vi "MIMICProtocol.vi"(4 "Input_Data":string[](array[string]), 5 "Error In":errorcluster, 6 "RSP_DelayTime":dbl caption="Delay Time (s)", 7 "ACK_DelayTime":dbl caption="Delay Time (s)", 8 "MIMIC_Command":string) -> (0 "Error Out":errorcluster, 1 "Status":bool, 2 "RESPONSE_Buffer":u8[](array[numeric]) format="%x", 3 "Generic_Mimic_Data 2":T1)   [LabVIEW 2014]
uses:
  Responses/MIMIC_ResponseCluster.ctl
panel:
  out "Validate \nCheckSum":bool
  out "ACK/NAK_Buffer":u8[](array[numeric])=[0, 0, 0, 0, 0, 0, 69, 83, 84, 32, 67, 79, 77, 80, 76, 69, 84, 69, 13, 10, 251, 226, 0, 0, 0, 0, 0, 0, 0, 0, 0, 0, 0, 0, 0, 0, 0, 0, 0, 0, 0, 0, 0, 0, 0, 0, 0, 0, 0, 0, 0, 0, 0, 0, 0, 0, 0, 0, 0, 0, 0, 0, 0, 0, 0, 0, 0, 0, 0, 0, 0, 0, 0, 0, 0, 0, 0, 0, 0, 0, 0, 0, 0, 0, 0, 0, 0, 0, 0, 0, 0, 0, 0, 0, 0, 0, 0, 0, 0, 0, 0, 0, 0, 0, 0, 0, 0, 0, 0, 0, 0, 0, 0, 0, 0, 0, 0, 0, 0, 0, 0, 0, 0, 0, 0, 0, 0, 0, 0, 0, 0, 0, 0, 0, 0, 0, 0, 0, 0, 0, 0, 0, 0, 0, 0, 0, 0, 0, 0, 0, 0, 0, 0, 0, 0, 0, 0, 0, 0, 0, 0, 0, 0, 0, 0, 0, 0, 0, 0, 0, 0, 0, 0, 0, 0, 0, 0, 0, 0, 0, 0, 0, 0, 0, 0, 0, 0, 0, 0, 0, 0, 0, 0, 0, 0, 0, 0, 0, 0, 0, 0, 0, 0, 0, 0, 0, 0, 0, 0, 0, 0, 0, 0, 0, 0, 0, 0, 0, 0, 0, 0, 0, 0, 0, 0, 0, 0, 0, 0, 0, 0, 0, 0, 0, 0, 0, 0, 0, 0, 0, 0, 0, 0, 0, 0, 0, 0, 0, 0, 0, 0, 0, 0, 0, 0, 0, 0, 0, 0, 0, 0, 0, 0, 0, 0, 0, 0, 0, 0, 0, 0, 0, 0, 0, 0, 0, 0] format="%x"
  in  "RSP_MimicProtocol VI Refnum":refnum<vi>
  out "Add \nChecksum":bool
  in  "CMD_MimicProtocol VI Refnum":refnum<vi>
  out "Send \nCommand":bool
  out "Command\n Sent":bool
  out "Response\n Received":bool
  out "ACK \nReceived":bool
  out "Check \nACK/NAK":bool
  out "Command":u8[](array[numeric]) format="%x"
  out "Obtain \nResponse":bool
  # "Outputs"
  # "Inputs"
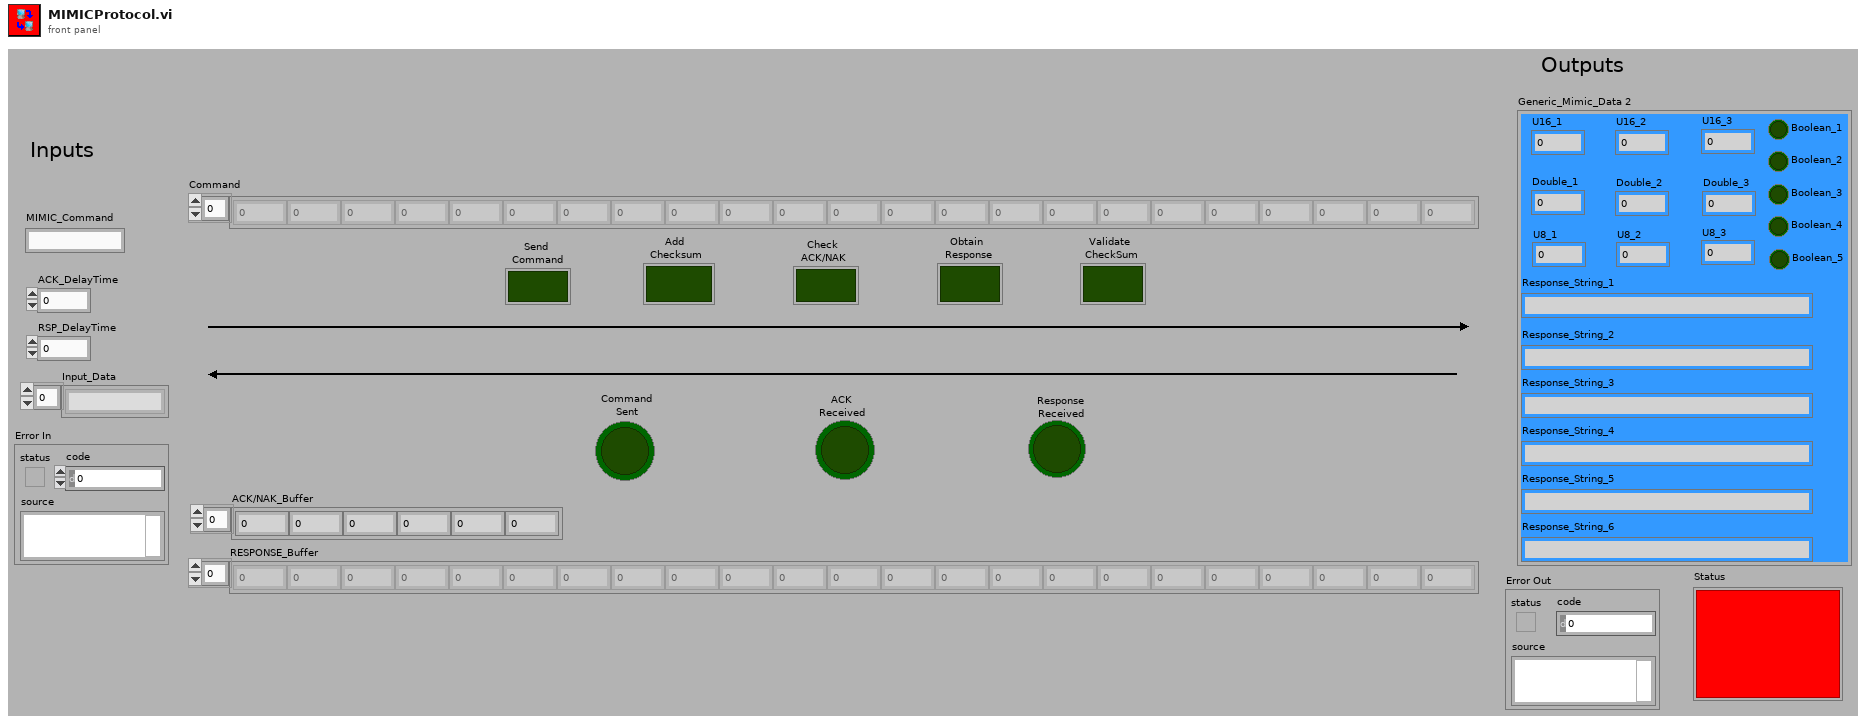
[diagram p1: front panel]
types:
  T1 = typedef "MIMIC_ResponseCluster.ctl" = cluster{"Response_String_1":string, "Response_String_2":string, "Response_String_3":string, "Response_String_4":string, "Response_String_5":string, "Response_String_6":string, "U16_1":u16, "Boolean_1":bool, "Boolean_2":bool, "Boolean_3":bool, "Boolean_4":bool, "Boolean_5":bool, "U16_2":u16, "U16_3":u16, "Double_1":dbl, "Double_2":dbl, "Double_3":dbl, "U8_1":dbl, "U8_2":dbl, "U8_3":dbl}
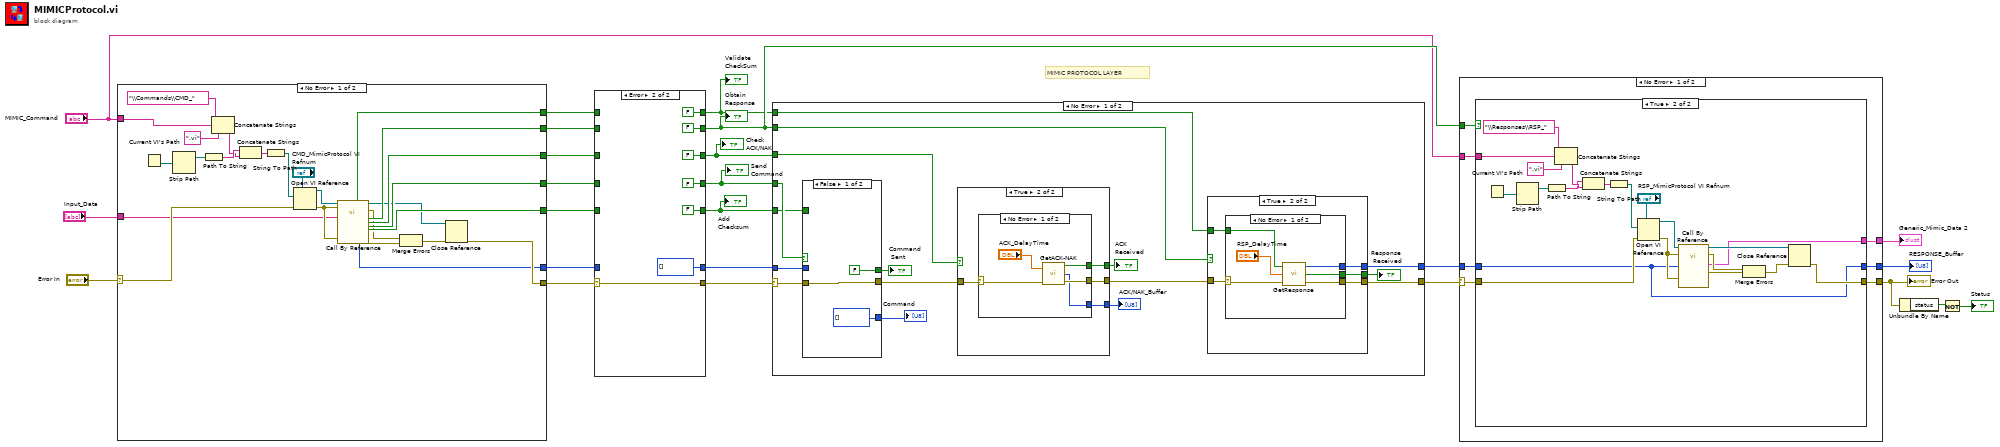
[diagram p0: block diagram]
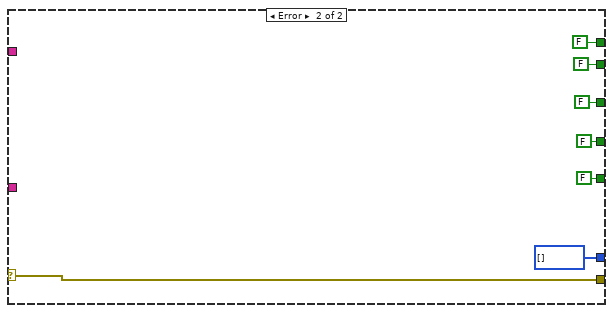
[diagram p3: hidden frame]
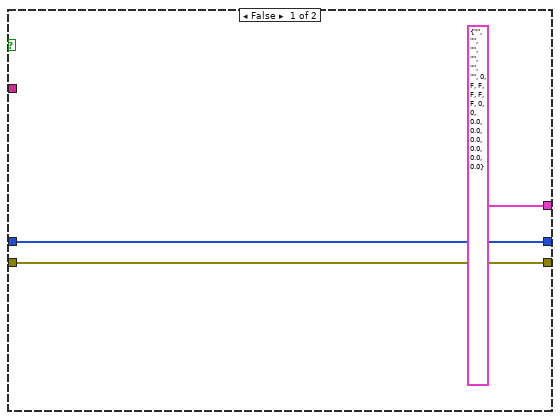
[diagram p4: hidden frame]
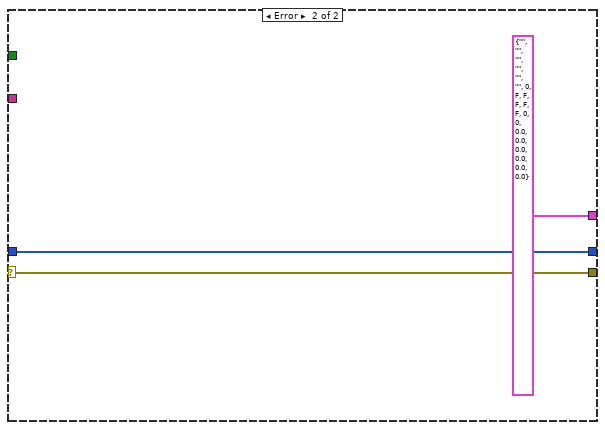
[diagram p5: hidden frame]
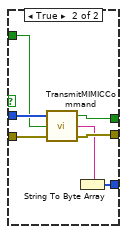
[diagram p6: hidden frame]
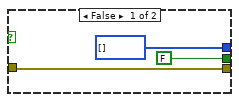
[diagram p7: hidden frame]
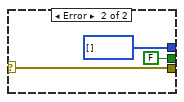
[diagram p8: hidden frame]
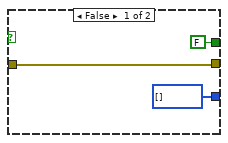
[diagram p9: hidden frame]
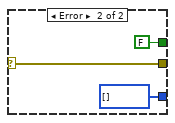
[diagram p10: hidden frame]
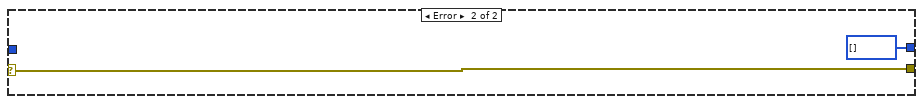
[diagram p11: hidden frame]
diagram:
  # "MIMIC PROTOCOL LAYER"
  n1 = case shown="No Error" "Error In" {
    selector: "Error In" -> [w48 w56]
    tunnel: [w43 w56] -> w12
    tunnel: "MIMIC_Command" -> [w46 _]
    tunnel: "Input_Data" -> [w34 _]
    tunnel: [w30 FALSE ("Command")] -> w16
    tunnel: [w31 FALSE ("Ack")] -> w18
    tunnel: [w32 FALSE ("Response")] -> w19
    tunnel: [w29 FALSE ("CheckSum")] -> w14
    tunnel: [w25 u8[] [] ("Command")] -> w10
    tunnel: [w28 FALSE ("Validate CheckSum")] -> w2
    frame No Error {
      n2 = Current VI's Path() -> (path=w49:path)
      n3 = Strip Path(path=w49) -> (stripped path=w42:path)  [unwired: 1 out]
      n4 = Path To String(path=w42) -> (string=w39:string)
      n5 = Concatenate Strings("\\Commands\\CMD_" ("string"), w46, ".vi" ("string")) -> (w38:string)
      n6 = Concatenate Strings(w39, w38) -> (w41:string)
      n7 = String To Path(string=w41) -> (path=w40:path)
      n8 = Open VI Reference(type specifier VI Refnum (for type only)="CMD_MimicProtocol VI Refnum", vi path=w40, error in (no error)=w48) -> (vi reference=w36:refnum<vi>, error out=w35:errorcluster)  [unwired: 3 in]
      n9 = call-by-ref "?"(reference=w36, error in=w35, "Input_Data"=w34, "Error In"=w35) -> (reference out=w26:refnum<vi>, error out=w27:errorcluster, "Validate CheckSum"=w28:bool, 13:"Command"=w25:u8[], "Response"=w32:bool, "Ack"=w31:bool, 16:"Command"=w30:bool, "Add CheckSum"=w29:bool, "Error Out"=w33:errorcluster)  [unwired: 10 in, 1 out]
      n10 = Merge Errors(w27, w33) -> (w44:errorcluster)
      n11 = Close Reference(reference=w26, error in (no error)=w44) -> (error out=w43:errorcluster)
    }
    frame Error {
    }
  }
  n12 = case shown="Error" w12 {
    selector: w12 -> [w59 w65]
    tunnel: [w63 FALSE ("Response")] -> w20
    tunnel: w19 -> [w63 _]
    tunnel: [w62 FALSE ("Ack")] -> w17
    tunnel: w18 -> [w62 _]
    tunnel: [w61 FALSE ("Command")] -> w15
    tunnel: w16 -> [w61 _]
    tunnel: [w60 FALSE ("CheckSum")] -> w13
    tunnel: w14 -> [w60 _]
    tunnel: [w59 w65] -> w11
    tunnel: [w58 u8[] [] ("Command")] -> w9
    tunnel: w10 -> [w58 _]
    tunnel: w2 -> [w57 _]
    tunnel: [w57 FALSE ("Validate CheckSum")] -> w1
    frame No Error {
    }
    frame Error {
    }
  }
  "Obtain \nResponse" <- w20
  "Check \nACK/NAK" <- w17
  "Send \nCommand" <- w15
  "Add \nChecksum" <- w13
  "Validate \nCheckSum" <- w1
  n13 = case shown="No Error" w11 {
    selector: w11 -> [w82 w130]
    tunnel: [w86 w130] -> w24
    tunnel: [w85 u8[] [] ("Receive_buffer out")] -> w23
    tunnel: w17 -> [w78 _]
    tunnel: w20 -> [w74 _]
    tunnel: w9 -> [w81 _]
    tunnel: w15 -> [w76 _]
    tunnel: w13 -> [w75 _]
    tunnel: w1 -> [w71 _]
    frame No Error {
      n14 = case shown="False" w76 {
        tunnel: [w89 w96] -> w84
        tunnel: w82 -> [w89 w95]
        tunnel: w81 -> [_ w94]
        tunnel: [FALSE ("Status") w93] -> w77
        tunnel: w75 -> [_ w92]
        tunnel: [u8[] [] ("unsigned byte array") w90] -> w72
        frame False {
        }
        frame True {
          n15 = call "TransmitMIMICCommand.vi"("Error In"=w95, "CheckSum?"=w92, "Command array"=w94) -> ("Error Out"=w96:errorcluster, "MIMIC_CMD"=w91:string, "Status"=w93:bool)
          n16 = String To Byte Array(string=w91) -> (unsigned byte array=w90:u8[])
        }
      }
      "Command\n Sent" <- w77
      "Command" <- w72
      n17 = case shown="True" w78 {
        tunnel: w84 -> [w116 w118]
        tunnel: [w116 w120] -> w83
        tunnel: [FALSE ("Status") w119] -> w80
        tunnel: [u8[] [] ("Receive_buffer") w117] -> w73
        frame False {
        }
        frame True {
          n18 = case shown="No Error" w118 {
            selector: w118 -> [w122 w128]
            tunnel: [w125 w128] -> w120
            tunnel: [w123 FALSE ("Status")] -> w119
            tunnel: [w121 u8[] [] ("Receive_buffer")] -> w117
            frame No Error {
              n19 = call "GetACK-NAK.vi"("error in"=w122, "Delay Time (s)"="ACK_DelayTime") -> ("error out"=w125:errorcluster, "Receive_buffer"=w121:u8[], "Status"=w123:bool)
            }
            frame Error {
            }
          }
        }
      }
      "ACK \nReceived" <- w80
      "ACK/NAK_Buffer" <- w73
      n20 = case shown="True" w74 {
        tunnel: [w99 w104] -> w86
        tunnel: [u8[] [] ("Receive_buffer out") w103] -> w85
        tunnel: w83 -> [w99 w101]
        tunnel: [FALSE ("Status") w102] -> w79
        tunnel: w71 -> [_ w100]
        frame False {
        }
        frame True {
          n21 = case shown="No Error" w101 {
            selector: w101 -> [w106 w113]
            tunnel: [w110 w113] -> w104
            tunnel: [w109 u8[] [] ("Receive_buffer out")] -> w103
            tunnel: [w107 FALSE ("Status")] -> w102
            tunnel: w100 -> [w105 _]
            frame No Error {
              n22 = call "GetResponse.vi"("error in"=w106, "Delay Time (s)"="RSP_DelayTime", "Validate Checksum"=w105) -> ("error out"=w110:errorcluster, "Status"=w107:bool, "Receive_buffer out"=w109:u8[])
            }
            frame Error {
            }
          }
        }
      }
      "Response\n Received" <- w79
    }
    frame Error {
    }
  }
  n23 = case shown="No Error" w24 {
    selector: w24 -> [w135 w162]
    tunnel: w23 -> [w136 w163]
    tunnel: w20 -> [w137 _]
    tunnel: [w134 w162] -> w7
    tunnel: [w133 w163] -> w8
    tunnel: "MIMIC_Command" -> [w132 _]
    tunnel: [w131 T1 {"Response_String_1"="", "Response_String_2"="", "Response_String_3"="", "Response_String_4"="", "Response_String_5"="", "Response_String_6"="", "U16_1"=0, "Boolean_1"=FALSE, "Boolean_2"=FALSE, "Boolean_3"=FALSE, "Boolean_4"=FALSE, "Boolean_5"=FALSE, "U16_2"=0, "U16_3"=0, "Double_1"=0.0, "Double_2"=0.0, "Double_3"=0.0, "U8_1"=0.0, "U8_2"=0.0, "U8_3"=0.0} ("Generic_Mimic_Data")] -> w3
    frame No Error {
      n24 = case shown="True" w137 {
        tunnel: w136 -> [w140 w142]
        tunnel: [w140 w142] -> w133
        tunnel: w135 -> [w139 w148]
        tunnel: [w139 w143] -> w134
        tunnel: w132 -> [_ w151]
        tunnel: [T1 {"Response_String_1"="", "Response_String_2"="", "Response_String_3"="", "Response_String_4"="", "Response_String_5"="", "Response_String_6"="", "U16_1"=0, "Boolean_1"=FALSE, "Boolean_2"=FALSE, "Boolean_3"=FALSE, "Boolean_4"=FALSE, "Boolean_5"=FALSE, "U16_2"=0, "U16_3"=0, "Double_1"=0.0, "Double_2"=0.0, "Double_3"=0.0, "U8_1"=0.0, "U8_2"=0.0, "U8_3"=0.0} ("Generic_Mimic_Data") w141] -> w131
        frame False {
        }
        frame True {
          n25 = Current VI's Path() -> (path=w152:path)
          n26 = Strip Path(path=w152) -> (stripped path=w156:path)  [unwired: 1 out]
          n27 = Path To String(path=w156) -> (string=w159:string)
          n28 = Concatenate Strings("\\Responses\\RSP_" ("string"), w151, ".vi" ("string")) -> (w160:string)
          n29 = Concatenate Strings(w159, w160) -> (w157:string)
          n30 = String To Path(string=w157) -> (path=w158:path)
          n31 = Open VI Reference(type specifier VI Refnum (for type only)="RSP_MimicProtocol VI Refnum", vi path=w158, error in (no error)=w148) -> (vi reference=w149:refnum<vi>, error out=w147:errorcluster)  [unwired: 3 in]
          n32 = call-by-ref "?"(reference=w149, error in=w147, "Error In"=w147, "Response"=w142) -> (reference out=w144:refnum<vi>, error out=w145:errorcluster, "Error Out"=w146:errorcluster, "Generic_Mimic_Data"=w141:T1)  [unwired: 1 out]
          n33 = Merge Errors(w145, w146) -> (w155:errorcluster)
          n34 = Close Reference(reference=w144, error in (no error)=w155) -> (error out=w143:errorcluster)
        }
      }
    }
    frame Error {
    }
  }
  "Error Out" <- w7
  "RESPONSE_Buffer" <- w8
  "Generic_Mimic_Data 2" <- w3
  n35 = Unbundle By Name(w7) -> ("status"=w6:bool)
  n36 = Not(x=w6) -> (.not. x?=→"Status":bool)
